vi "Untitled 6.vi"() -> ()   [LabVIEW 2015]
panel:
  in  "Load From File":bool
  in  "Save To File":bool
  in  "Clear Last Value":bool
  in  "Clear Graph":bool
  in  "Get Vol":bool
  in  "stop":bool
  out "Data":cluster{dbl[], dbl[]}[](array[cluster])
  in  "VISA resource name":refnum<visa-resource-name>="VAL_N6705B"
  out "XY Graph":cluster{dbl[], dbl[]}[](graph)
  in  "Delay(ms)":u16
  in  "N":u16
  in  "Step":dbl
  in  "Start":dbl
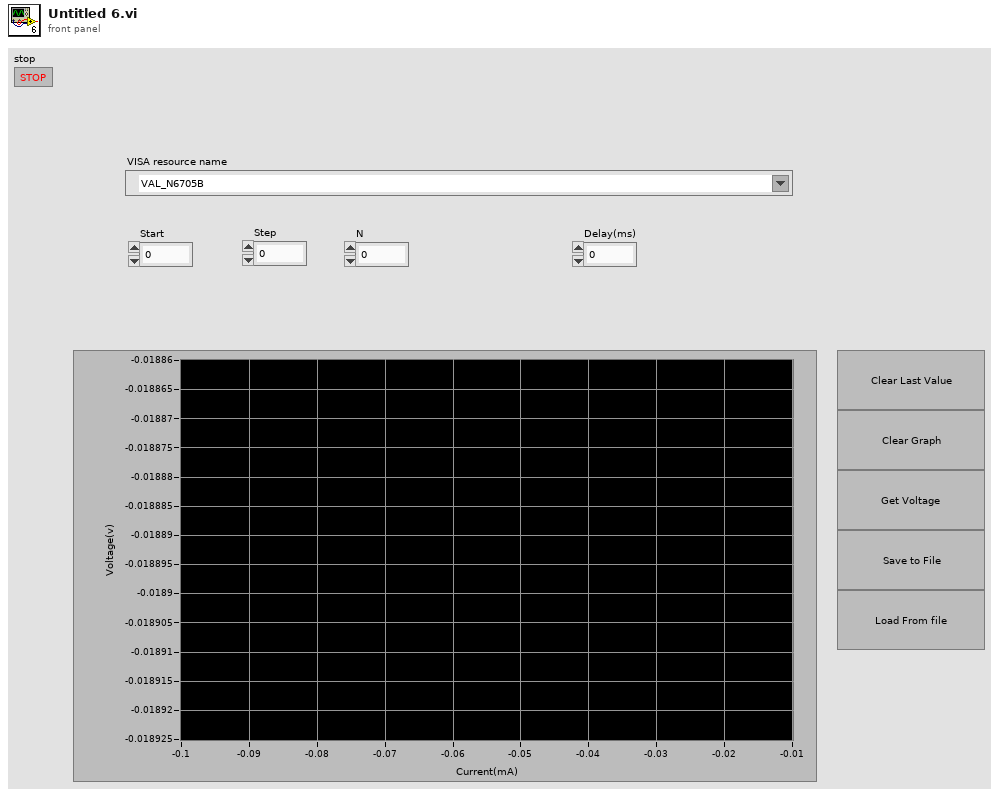
[diagram p1: front panel]
types:
  T1 = enum16{"open", "replace", "create", "open or create", "replace or create", "replace or create with confirmation"}
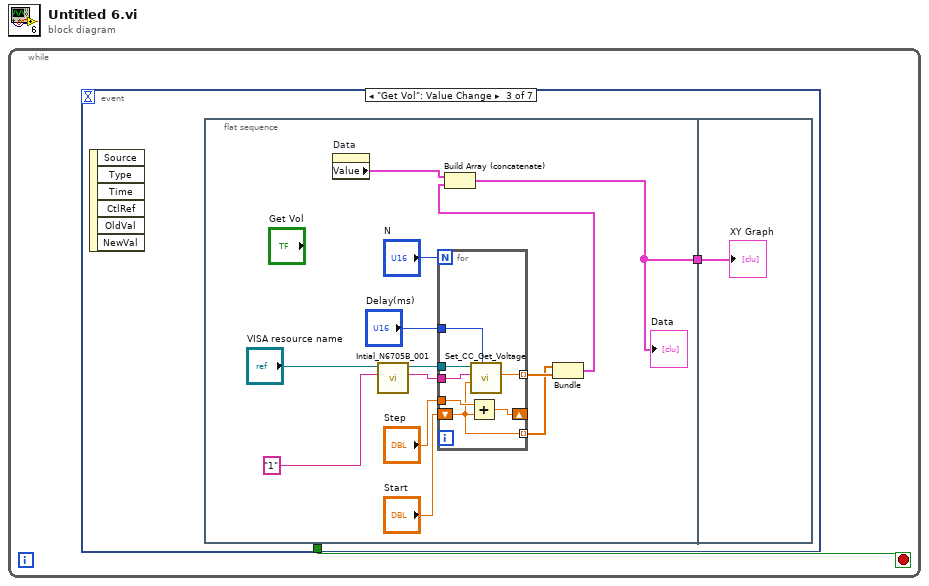
[diagram p0: block diagram]
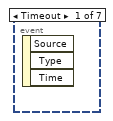
[diagram p2: hidden frame]
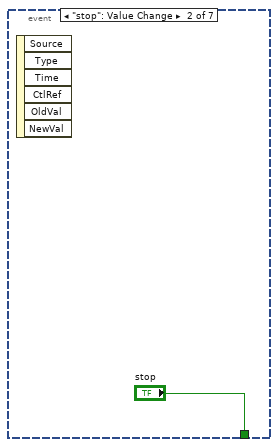
[diagram p3: hidden frame]
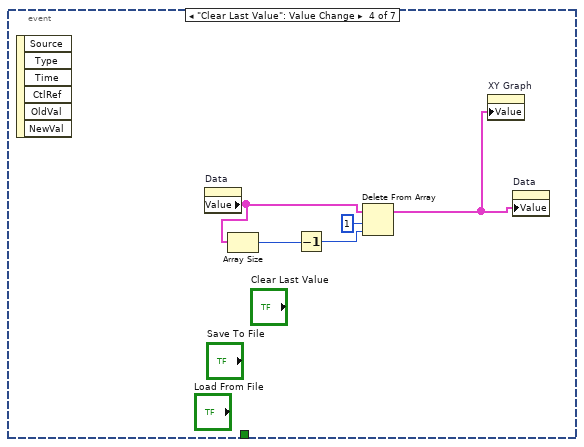
[diagram p4: hidden frame]
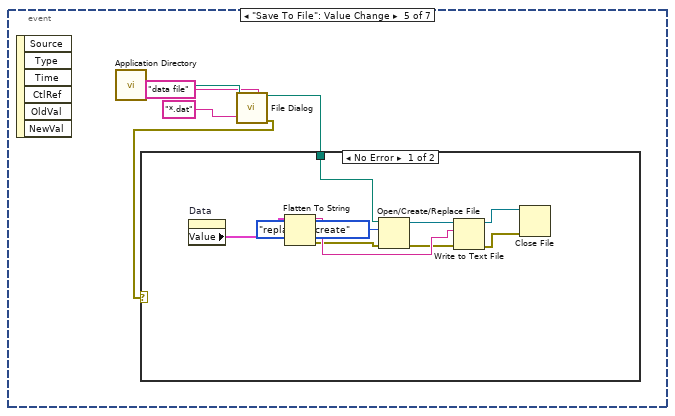
[diagram p5: hidden frame]
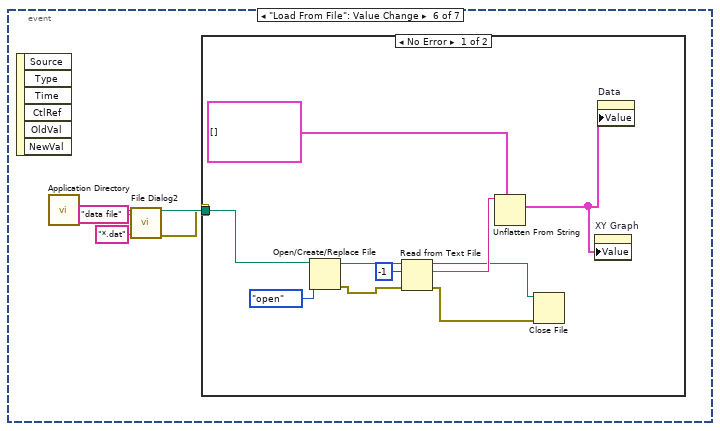
[diagram p7: hidden frame]
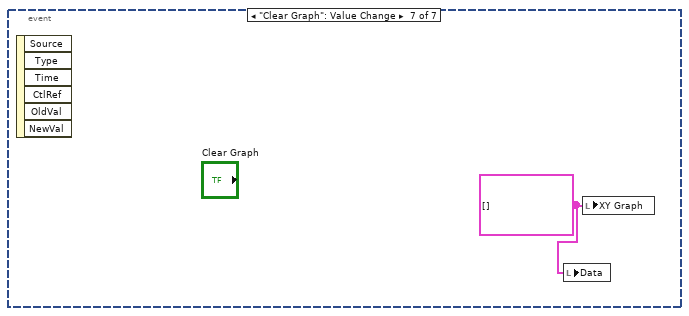
[diagram p9: hidden frame]
diagram:
  n1 = while {
    stop <- w1 stop-if-true
    n2 = event shown="[2] \"Get Vol\": Value Change" {
      selector: _ -> [_ _ _ _ _ _ _]
      dyn-events: _ -> [_ _ _ _ _ _ _]
      timeout: _ -> [_ _ _ _ _ _ _]
      tunnel: [_ "stop" _ _ _ _ _] -> w1
      event Timeout {
        n3 = event-data() -> ()  [unwired: 1 in, 3 out]
      }
      event "stop": Value Change {
        n4 = event-data() -> ()  [unwired: 1 in, 6 out]
      }
      event "Get Vol": Value Change {
        n5 = event-data() -> ()  [unwired: 1 in, 6 out]
        n6 = flat-sequence {
          tunnel: [w4] -> w3
          tunnel: w3 -> [w24]
          frame #0 {
            n7 = property on="Data" class="Arr (strict)"() -> ("Value"=w6:cluster{dbl[], dbl[]}[])  [unwired: 2 in, 2 out]
            n8 = call "Intial_N6705B_001.vi"("Channel Name (1) in"="1" ("Channel Name (1)"), "VISA Refnum in"="VISA resource name") -> ("Channel Name (1) out"=w14:string, "VISA Refnum out"=w13:refnum<visa-resource-name>)  [unwired: 7 in, 1 out]
            n9 = for {
              N: "N" -> [_]
              tunnel: "Step" -> [w19]
              tunnel: "Delay(ms)" -> [w23]
              tunnel: w13 -> [w22]
              tunnel: w14 -> [w21]
              shift-right: [w20] -> _
              shift-left: "Start" -> [w18]
              tunnel: [w18] -> w15 mode=indexing
              tunnel: [w17] -> w16 mode=indexing
              n10 = Add(x=w19, y=w18) -> (x+y=w20:dbl)
              n11 = call "Set_CC_Get_Voltage.vi"("Delay to Measure"=w23, "Limit (1.0 A)"=w18, "Channel Name (1)"=w21, "VISA Refnum in"=w22) -> ("Voltage Measurement"=w17:dbl)  [unwired: 4 in, 3 out]
            }
            n12 = Bundle(w15, w16) -> (w5:cluster{dbl[], dbl[]})  [unwired: 1 in]
            n13 = Build Array (concatenate)(w6, w5) -> (w4:cluster{dbl[], dbl[]}[])
            "Data" <- w4
          }
          frame #1 {
            "XY Graph" <- w24
          }
        }
      }
      event "Clear Last Value": Value Change {
        n14 = event-data() -> ()  [unwired: 1 in, 6 out]
        n15 = property on="Data" class="Arr (strict)"() -> ("Value"=w28:cluster{dbl[], dbl[]}[])  [unwired: 2 in, 2 out]
        n16 = Array Size(array=w28) -> (size(s)=w26:i32)
        n17 = Decrement(x=w26) -> (x-1=w25:i32)
        n18 = Delete From Array(array=w28, length=1, index=w25) -> (array with subset deleted=w27:cluster{dbl[], dbl[]}[])  [unwired: 1 out]
        n19 = property on="XY Graph" class="XYGraph (strict)"("Value"=w27) -> ()  [unwired: 2 in, 2 out]
        n20 = property on="Data" class="Arr (strict)"("Value"=w27) -> ()  [unwired: 2 in, 2 out]
      }
      event "Save To File": Value Change {
        n21 = event-data() -> ()  [unwired: 1 in, 6 out]
        n22 = call <vilib>:"Application Directory.vi"() -> ("Application Directory"=w34:path)
        n23 = call "File Dialog"("start path"=w34, "pattern (all files)"="*.dat", "pattern label"="data file") -> ("selected path"=w31:path, "error out"=w30:errorcluster)  [unwired: 9 in, 2 out]
        n24 = case shown="No Error" w30 {
          tunnel: w31 -> [w42 _]
          frame No Error {
            n25 = property on="Data" class="Arr (strict)"() -> ("Value"=w43:cluster{dbl[], dbl[]}[])  [unwired: 2 in, 2 out]
            n26 = Flatten To String(anything=w43) -> (data string=w40:string, error out=w39:errorcluster)  [unwired: 3 in, 1 out]
            n27 = Open/Create/Replace File(file path (use dialog)=w42, error in=w39, operation (0:open)=T1."replace or create") -> (refnum out=w41:refnum<file>, error out=w38:errorcluster)  [unwired: 3 in, 1 out]
            n28 = Write to Text File(file (use dialog)=w41, text=w40, error in=w38) -> (refnum out=w37:refnum<file>, error out=w36:errorcluster)  [unwired: 1 in, 1 out]
            n29 = Close File(refnum=w37, error in=w36) -> ()  [unwired: 2 out]
          }
          frame Error {
          }
        }
      }
      event "Load From File": Value Change {
        n30 = event-data() -> ()  [unwired: 1 in, 6 out]
        n31 = call <vilib>:"Application Directory.vi"() -> ("Application Directory"=w48:path)
        n32 = call "File Dialog2"("start path"=w48, "pattern (all files)"="*.dat", "pattern label"="data file") -> ("selected path"=w45:path, "error out"=w44:errorcluster)  [unwired: 9 in, 2 out]
        n33 = case shown="No Error" w44 {
          tunnel: w45 -> [w58 _]
          frame No Error {
            n34 = Open/Create/Replace File(file path (use dialog)=w58, operation (0:open)=T1."open") -> (refnum out=w56:refnum<file>, error out=w54:errorcluster)  [unwired: 4 in, 1 out]
            n35 = Read from Text File(file (use dialog)=w56, count=-1, error in=w54) -> (refnum out=w50:refnum<file>, text=w53:string, error out=w49:errorcluster)  [unwired: 1 in, 1 out]
            n36 = Unflatten From String(type=cluster{dbl[], dbl[]}[] [] ("Data"), binary string=w53) -> (value=w51:cluster{dbl[], dbl[]}[])  [unwired: 3 in, 2 out]
            n37 = Close File(refnum=w50, error in=w49) -> ()  [unwired: 2 out]
            n38 = property on="XY Graph" class="XYGraph (strict)"("Value"=w51) -> ()  [unwired: 2 in, 2 out]
            n39 = property on="Data" class="Arr (strict)"("Value"=w51) -> ()  [unwired: 2 in, 2 out]
          }
          frame Error {
          }
        }
      }
      event "Clear Graph": Value Change {
        w59 = cluster{dbl[], dbl[]}[] [] ("XY Graph")
        n40 = event-data() -> ()  [unwired: 1 in, 6 out]
        n41 = local write "Data"(w59) -> ()
        n42 = local write "XY Graph"(w59) -> ()
      }
    }
  }
